vi "InitCfg.vi"(8 "error in (no error)":errorcluster, 11 "Cfg File path":path=path "C:/Users/Public/Documents/OU PAARD/mmWave_RF_Scanner/SupportFiles/mmWaveConfig.ini") -> (0 "error out":errorcluster, 3 "aparCfg out":refnum<class "aparCfg.lvclass">)   [LabVIEW 2018, in "aparCfg.lvclass"]
uses:
  aparCfg.lvclass
  aparConfig.ctl
  N5222A PNA/N5222AConfig.ctl
  ArrayController/ACConfig.ctl
  Datalog/DataLogConfig.ctl
  aparCfg.lvclass/aparCfg.ctl
panel:
  in  "apar properties":T1={"N5222AConfig"={"ResourceName"="PNA", "Enable"=FALSE, "Channel"=1, "CalFileName"="", "MeasName"="", "TempDatFile"="", "Power, dBm"=-30.0, "NumPoints"=201, "Start Freq, Hz"=5000000000.0, "Stop Freq, Hz"=6000000000.0, "NumAverages"=20, "Sweep Type"=0}, "ACConfig"={"Board 1 alias"="AO-1/ao0:31", "Board 1 Enable"=FALSE, "Board 2 alias"="AO-2/ao0:31", "Board 2 Enable"=FALSE}, "DataLogConfig"={"FilePath"=path ""}} {"N5222AConfig"."Sweep Type" items=["Linear Frequency", "Log Frequency", "Power Sweep", "CW Time"]; "N5222AConfig"."Stop Freq, Hz" format="%_3p"; "N5222AConfig"."Start Freq, Hz" format="%_3p"}
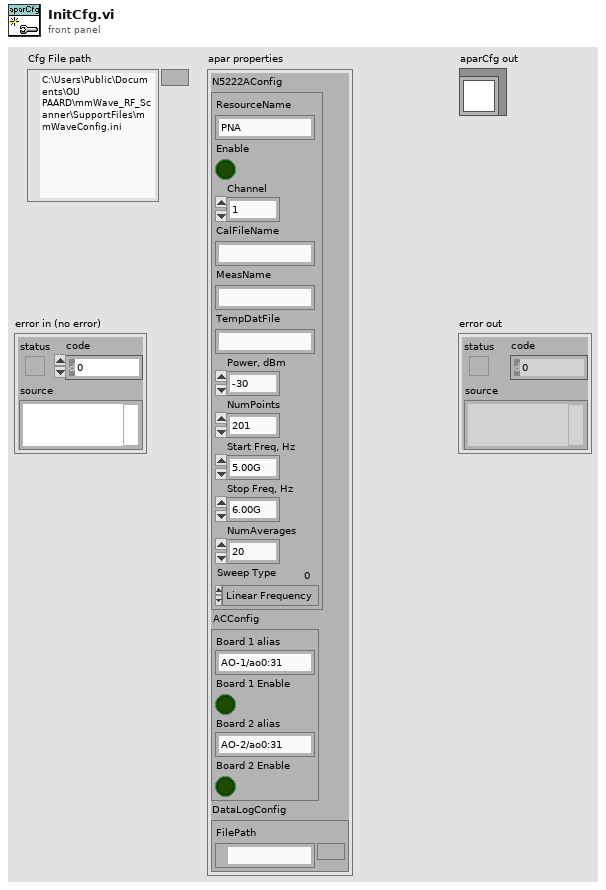
[diagram p1: front panel]
types:
  T1 = typedef "aparCfg.lvclass/aparConfig.ctl" = cluster{"N5222AConfig":T2, "ACConfig":T3, "DataLogConfig":T4}
  T2 = typedef "N5222AConfig.ctl" = cluster{"ResourceName":string, "Enable":bool, "Channel":i32, "CalFileName":string, "MeasName":string, "TempDatFile":string, "Power, dBm":dbl, "NumPoints":i32, "Start Freq, Hz":dbl, "Stop Freq, Hz":dbl, "NumAverages":i32, "Sweep Type":i32}
  T3 = typedef "ACConfig.ctl" = cluster{"Board 1 alias":string, "Board 1 Enable":bool, "Board 2 alias":string, "Board 2 Enable":bool}
  T4 = typedef "DataLogConfig.ctl" = cluster{"FilePath":path}
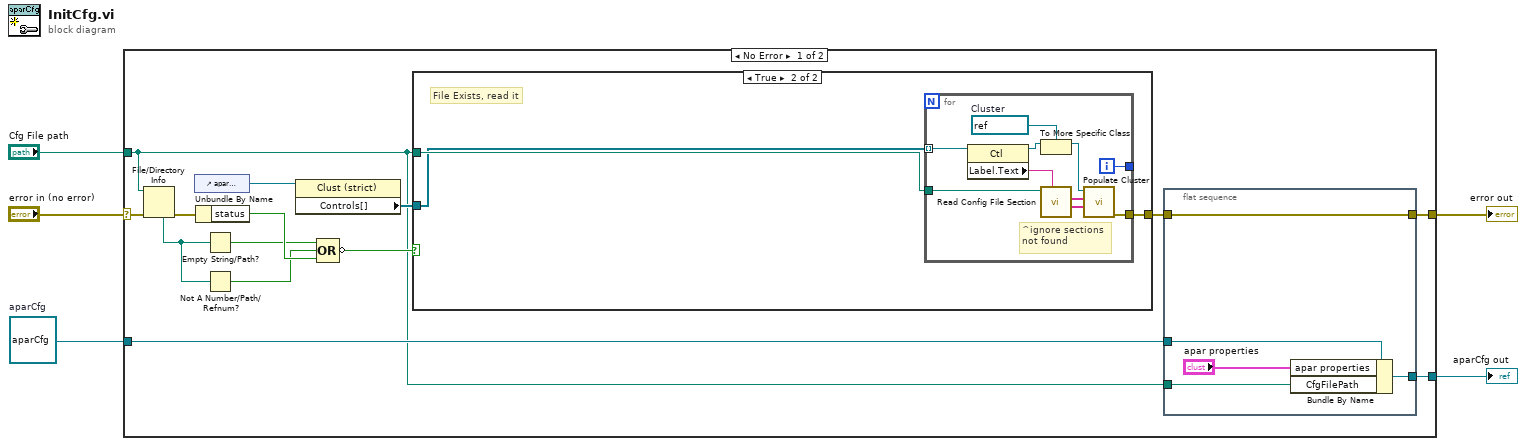
[diagram p0: block diagram]
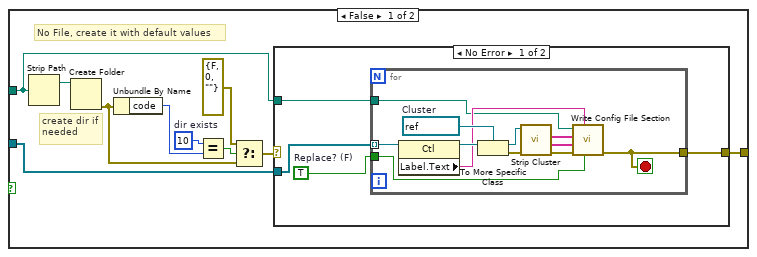
[diagram p2: hidden frame]
diagram:
  w4 = refnum<class "aparCfg.lvclass"> refnum  # aparCfg
  n1 = case shown="No Error" "error in (no error)" {
    selector: "error in (no error)" -> [w9 w66]
    tunnel: [w8 w66] -> w2
    tunnel: [w10 w65] -> w1
    tunnel: w4 -> [w11 w65]
    tunnel: "Cfg File path" -> [w7 _]
    frame No Error {
      n2 = File/Directory Info(path=w7, error in=w9) -> (error out=w15:errorcluster, resolved path=w12:path)  [unwired: 5 out]
      n3 = control-ref of="apar properties"() -> (w6:refnum<vi>)
      n4 = Unbundle By Name(w15) -> ("status"=w16:bool)
      n5 = Empty String/Path?(string/path=w12) -> (empty?=w13:bool)
      n6 = Not A Number/Path/Refnum?(number/path/refnum=w12) -> (NaN/Path/Refnum?=w14:bool)
      n7 = property class="Clust (strict)"(reference=w6) -> ("Controls[]"=w17:refnum<vi>[])  [unwired: 1 in, 2 out]
      n8 = Compound Arithmetic op=OR(w13, w14, w16) -> (invert w18:bool)
      n9 = case shown="True" w18 {
        tunnel: w7 -> [w32 w54]
        tunnel: w17 -> [w34 w53]
        tunnel: [w33 w52] -> w19
        frame False {
          w27 = 10  # dir exists
          # "create dir if\nneeded"
          # "No File, create it with default values"
          n10 = Strip Path(path=w32) -> (stripped path=w29:path)  [unwired: 1 out]
          n11 = Create Folder(path (use dialog)=w29) -> (error out=w28:errorcluster)  [unwired: 2 in, 2 out]
          n12 = Unbundle By Name(w28) -> ("code"=w31:i32)
          n13 = Equal?(x=w27, y=w31) -> (x = y?=w30:bool)
          n14 = Select(t=errorcluster {"status"=FALSE, "code"=0, "source"=""}, s=w30, f=w28) -> (s? t:f=w25:errorcluster)
          n15 = case shown="No Error" w25 {
            selector: w25 -> [_ w51]
            tunnel: w34 -> [w38 _]
            tunnel: [w36 w51] -> w33
            tunnel: w32 -> [w35 _]
            frame No Error {
              w37 = TRUE  # Replace? (F)
              n16 = for {
                tunnel: w38 -> [w43] mode=indexing
                tunnel: [w44] -> w36
                tunnel: w37 -> [w40]
                tunnel: w35 -> [w39]
                stop <- w44 stop-if-true
                w50 = refnum<vi> refnum  # Cluster
                n17 = property class="Ctl"(reference=w43) -> (reference out=w42:refnum<vi>, "Label.Text"=w41:string)  [unwired: 1 in, 1 out]
                n18 = To More Specific Class(target class=w50, reference=w42) -> (specific class reference=w49:refnum<vi>, error out=w46:errorcluster)  [unwired: 1 in]
                n19 = call "Strip Cluster.vi"("error in (no error)"=w46, "Cluster Refnum"=w49) -> ("error out"=w45:errorcluster, "Values"=w47:string[], "Keys"=w48:string[])  [unwired: 6 in, 1 out]
                n20 = call "Write Config File Section.vi"("Replace? (F)"=w40, "Section"=w41, "error in"=w45, "Values"=w47, "Keys"=w48, "INI path"=w39) -> ("error out"=w44:errorcluster)  [unwired: 5 in]
              }
            }
            frame Error {
            }
          }
        }
        frame True {
          # "File Exists, read it"
          n21 = for {
            tunnel: w53 -> [w64] mode=indexing
            tunnel: w54 -> [w62]
            tunnel: [w59] -> w52
            tunnel: [w55] -> _
            i -> [w55]
            w58 = refnum<vi> refnum  # Cluster
            # "^ignore sections\nnot found"
            n22 = property class="Ctl"(reference=w64) -> (reference out=w57:refnum<vi>, "Label.Text"=w63:string)  [unwired: 1 in, 1 out]
            n23 = To More Specific Class(target class=w58, reference=w57) -> (specific class reference=w56:refnum<vi>)  [unwired: 1 in, 1 out]
            n24 = call "Read Config File Section.vi"("Section"=w63, "appended path"=w62) -> ("Values"=w60:string[], "Keys"=w61:string[])  [unwired: 7 in, 1 out]
            n25 = call "Populate Cluster.vi"("Values"=w60, "Keys"=w61, "Clust Refnum"=w56) -> ("error out"=w59:errorcluster)  [unwired: 7 in, 1 out]
          }
        }
      }
      n26 = flat-sequence {
        tunnel: w7 -> [w24]
        tunnel: w11 -> [w23]
        tunnel: [w22] -> w10
        tunnel: [w21] -> w8
        tunnel: w19 -> [w21]
        frame #0 {
          n27 = Bundle By Name(cluster=w23, "apar properties"="apar properties", "CfgFilePath"=w24) -> (w22:refnum<class "aparCfg.lvclass">)
        }
      }
    }
    frame Error {
    }
  }
  "error out" <- w2
  "aparCfg out" <- w1
